vi "Set Shutter.vi"(8 "error in (no error)":errorcluster, 11 "CCDCamera in":refnum<class "CCDCamera.lvclass">) -> (0 "error out":errorcluster, 3 "CCDCamera out":refnum<class "CCDCamera.lvclass">)   [LabVIEW 2018, in "CCDCamera.lvclass"]
uses:
  CCDCamera.lvclass
  C:/Users/observer/Desktop/SPARC4_ACS/SPARC4_ACS/Simulated_CCD_Camera/Simulated_CCD_Camera.lvclass
  Simulated_CCD_Camera/Simulated_CCD_Camera.lvclass/Simulated_CCD_Camera.ctl
  Interface/Interface.lvclass/Interface.ctl
  Interface/Interface.lvclass
  Simulated_CCD_Camera/Simulated_CCD_Camera.lvclass
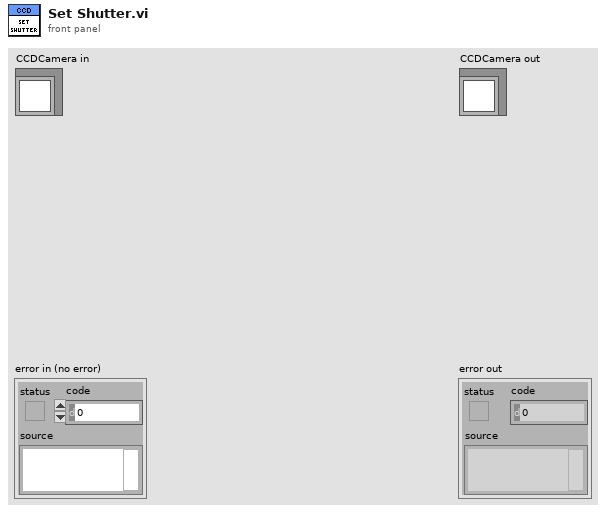
[diagram p1: front panel]
types:
  T1 = typedef "Shutter_mode typedef.ctl" = enum16{"Auto", "Open", "Close", "N/A (3)", "Open FVB Series", "Open Any Series"}
  T2 = typedef "ReadMode_mode typedef.ctl" = enum16{"Full Vertical Binning", "Multi-Track", "Random-Track", "Single-Track", "Image"}
  T3 = typedef "AcquisitionMode_mode typedef.ctl" = enum16{"Reserved (0)", "Single Scan", "Accumulate", "Kinetics", "Fast Kinetics", "Run Till Abort", "Reserved (6)", "Reserved (7)", "Reserved (8)", "Time Delayed Integration"}
  T4 = cluster{"EXPTIME":sgl, "PREAMP":enum16{"Gain 1", "Gain 2"}, "READOUT_RATE":enum16{"30 MHz", "20 MHz", "10 MHz", "1 MHz"}, "EM_GAIN":u16, "VBIN":u16, "INITIAL_LINE":u16, "INITIAL_COLUMN":u16, "FINAL_LINE":u16, "FINAL_COLUMN":u16, "#FRAMES":u32, "#CUBES":u32, "TRIGGER_MODE":enum16{"Internal", "External", "N/A", "N/A_1", "N/A_2", "N/A_3", "External Start"}, "HBIN":u16, "SHUTTER_TTL":enum16{"TTL Low", "TTL High"}, "SHUTTER_MODE":T1, "SHUTTER_OPENING_TIME":u16, "SHUTTER_CLOSING_TIME":u16, "VERTICAL_SHIFT_SPEED":u16, "READ_MODE":T2, "FRAME_TRANSFER":bool, "VERTICAL_CLOCK_VOLTAGE":enum16{"0", "+1", "+2", "+3", "+4"}, "ACQUISITION_MODE":T3, "AD_CHANNEL":u16, "EM_MODE":enum16{"Electron Multiplying", "Conventional"}, "Error In":errorcluster}
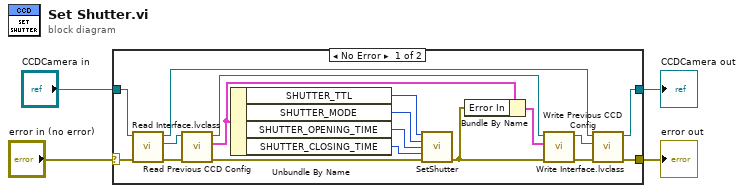
[diagram p0: block diagram]
diagram:
  n1 = case shown="No Error" "error in (no error)" {
    selector: "error in (no error)" -> [w21 w24]
    tunnel: [w9 w24] -> w3
    tunnel: [w10 w23] -> w1
    tunnel: "CCDCamera in" -> [w22 w23]
    frame No Error {
      n2 = call "Read Interface.lvclass.vi"("error in (no error)"=w21, "Simulated_CCD_Camera in"=w22) -> ("error out"=w15:errorcluster, "Interface.lvclass"=w20:refnum<class "Interface.lvclass">, "Simulated_CCD_Camera out"=w8:refnum<class "CCDCamera.lvclass">)  [unwired: 7 in]
      n3 = call "Read Previous CCD Config.vi"("error in (no error)"=w15, "Interface in"=w20) -> ("error out"=w14:errorcluster, "Previous CCD Config"=w13:T4, "Interface out"=w5:refnum<class "Interface.lvclass">)  [unwired: 7 in]
      n4 = Unbundle By Name(w13) -> ("SHUTTER_TTL"=w19:enum16{"TTL Low", "TTL High"}, "SHUTTER_MODE"=w18:T1, "SHUTTER_OPENING_TIME"=w17:u16, "SHUTTER_CLOSING_TIME"=w16:u16)
      n5 = call <userlib>:"SetShutter.vi"("type"=w19, "mode"=w18, "closingtime"=w17, "openingtime"=w16, "error in (no error)"=w14) -> ("error out"=w6:errorcluster)  [unwired: 9 in, 1 out]
      n6 = Bundle By Name(cluster=w13, "Error In"=w6) -> (w12:T4)
      n7 = call "Write Previous CCD Config.vi"("error in (no error)"=w6, "Previous CCD Config"=w12, "Interface in"=w5) -> ("error out"=w7:errorcluster, "Interface out"=w11:refnum<class "Interface.lvclass">)  [unwired: 7 in]
      n8 = call "Write Interface.lvclass.vi"("error in (no error)"=w7, "Interface.lvclass"=w11, "Simulated_CCD_Camera in"=w8) -> ("error out"=w9:errorcluster, "Simulated_CCD_Camera out"=w10:refnum<class "CCDCamera.lvclass">)  [unwired: 7 in]
    }
    frame Error {
    }
  }
  "error out" <- w3
  "CCDCamera out" <- w1
